vi "Array Max & Min Numeric Value.vi"(7 "JSON Value in":refnum<class "JSON Value.lvclass">, 11 "error in (no error)":errorcluster) -> (4 "max value":dbl, 6 "max index":i32, 8 "min value":dbl, 10 "min index":i32, 15 "error out":errorcluster)   [LabVIEW 2016, in "JSON Value.lvclass"]
uses:
  JSON Helper/JSON Value.lvclass
  JSON Numeric/Read value (Numeric).vi
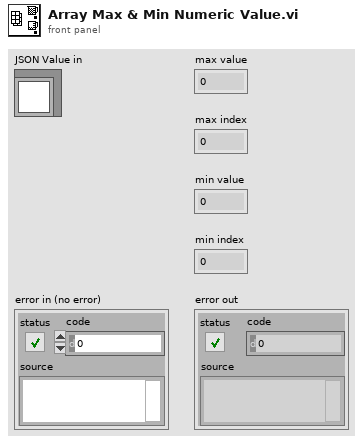
[diagram p1: front panel]
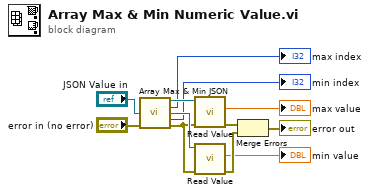
[diagram p0: block diagram]
diagram:
  n1 = call "Array Max & Min JSON.vi"("JSON Value in"="JSON Value in", "error in (no error)"="error in (no error)") -> (4:"JSON Value out"=w10:refnum<class "JSON Value.lvclass">, "max index"=→"max index":i32, 8:"JSON Value out"=w9:refnum<class "JSON Value.lvclass">, "min index"=→"min index":i32, "error out"=w3:errorcluster)  [unwired: 9 in]
  n2 = call-poly "Read Value.vi"("error in (no error)"=w3, "JSON Value in"=w10) -> ("error out"=w6:errorcluster, "value"=→"max value":dbl)  [unwired: 8 in]
  n3 = call-poly "Read Value.vi"("error in (no error)"=w3, "JSON Value in"=w9) -> ("error out"=w5:errorcluster, "value"=→"min value":dbl)  [unwired: 8 in]
  n4 = Merge Errors(w6, w5) -> (→"error out":errorcluster)
